vi "Configure.vi"(8 "error in (no error)":errorcluster, 10 "DisableRTProtocol":bool) -> (0 "error out":errorcluster, 2 "reboot required":bool)   [LabVIEW 2017, in "RTProtocol.lvlib"]
uses:
  <vilib>/addons/InsightCM/Utilities/Security/RTProtocol/RTProtocol.lvlib
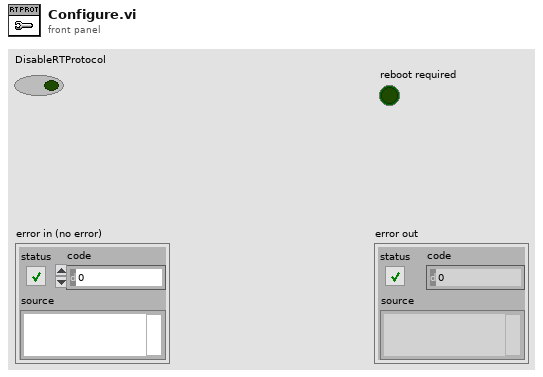
[diagram p1: front panel]
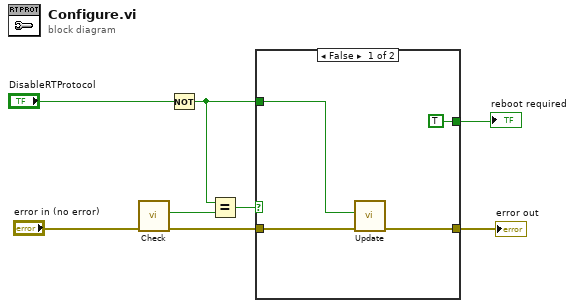
[diagram p0: block diagram]
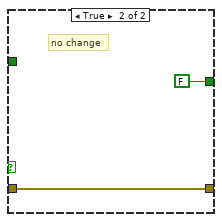
[diagram p2: hidden frame]
diagram:
  n1 = call <vilib>:"Check.vi"("error in (no error)"="error in (no error)") -> ("error out"=w5:errorcluster, "enabled"=w6:bool)  [unwired: 9 in]
  n2 = Not(x="DisableRTProtocol") -> (.not. x?=w3:bool)
  n3 = Equal?(x=w3, y=w6) -> (x = y?=w4:bool)
  n4 = case shown="False" w4 {
    tunnel: w5 -> [w12 w14]
    tunnel: [w11 w14] -> w2
    tunnel: w3 -> [w10 _]
    tunnel: [TRUE FALSE] -> w1
    frame False {
      n5 = call <vilib>:"Update.vi"("error in (no error)"=w12, "enable"=w10) -> ("error out"=w11:errorcluster)  [unwired: 9 in]
    }
    frame True {
      # "no change"
    }
  }
  "error out" <- w2
  "reboot required" <- w1
